vi "DecodeTriggerSettings.vi"(8 "error in (no error)":errorcluster, 9 "ParameterLabel":string, 10 "Arg":string, 11 "Highland T564 DDG in":refnum<class "Highland T564 DDG.lvclass">) -> (0 "error out":errorcluster, 3 "Highland T564 DDG out":refnum<class "Highland T564 DDG.lvclass">)   [LabVIEW 2020, in "Highland T564 DDG.lvclass"]
uses:
  Highland T564 DDG.lvclass
  C:/GEECS/Developers Version/source/Device Drivers/shared/MetaDriver_v1/MetaDriver_v1.lvclass
  shared/Typdefs/Choice81.ctl
  shared/Typdefs/Choice82.ctl
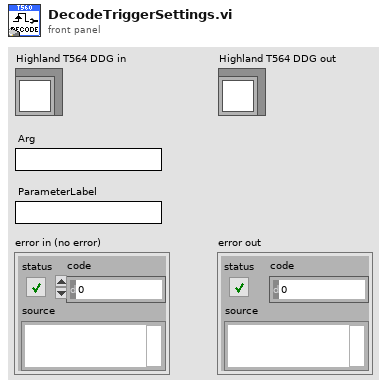
[diagram p1: front panel]
types:
  T1 = typedef "Choice81.ctl" = enum16{"10KOhm", "50Ohms"}
  T2 = typedef "Choice82.ctl" = enum16{"Rising", "Falling", "Internal 80MHz", "Internal DDS", "Remote", "Disabled"}
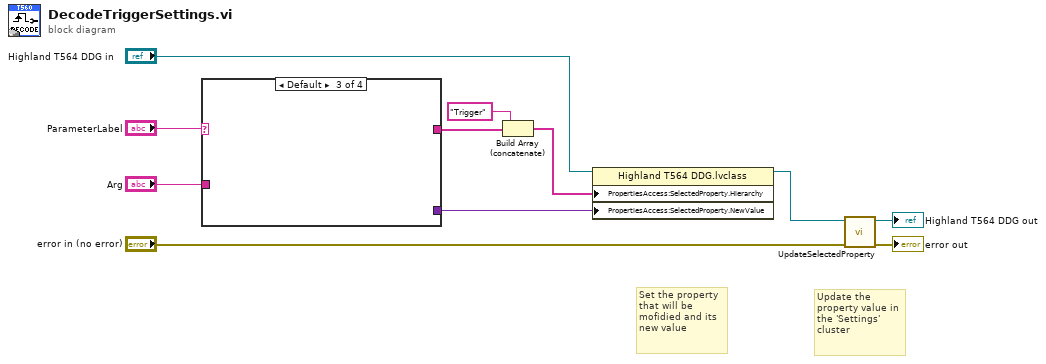
[diagram p0: block diagram]
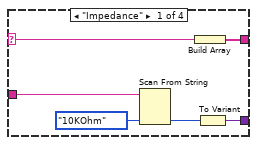
[diagram p2: hidden frame]
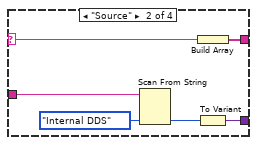
[diagram p3: hidden frame]
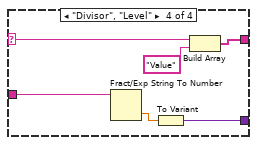
[diagram p4: hidden frame]
diagram:
  # "Update the property value in the 'Settings' cluster"
  # "Set the property that will be mofidied and its new value"
  n1 = case shown="Default" "ParameterLabel" {
    selector: "ParameterLabel" -> [w17 w23 _ w26]
    tunnel: "Arg" -> [w15 w21 _ w29]
    tunnel: [w13 w19 _ w28] -> w5
    tunnel: [w12 w18 _ w24] -> w11
    frame "Impedance" {
      n2 = Scan From String(input string=w15, default 1=Choice81."10KOhm" ("Polarity")) -> (output 1=w14:T1)  [unwired: 3 in, 3 out]
      n3 = Build Array(w17) -> (w12:string[])
      n4 = To Variant(anything=w14) -> (Variant=w13:variant)
    }
    frame "Source" {
      n5 = Scan From String(input string=w21, default 1=Choice82."Internal DDS" ("ON/OFF")) -> (output 1=w20:T2)  [unwired: 3 in, 3 out]
      n6 = Build Array(w23) -> (w18:string[])
      n7 = To Variant(anything=w20) -> (Variant=w19:variant)
    }
    frame Default {
    }
    frame "Divisor", "Level" {
      n8 = Fract/Exp String To Number(string=w29) -> (number=w27:dbl)  [unwired: 3 in, 1 out]
      n9 = To Variant(anything=w27) -> (Variant=w28:variant)
      n10 = Build Array(w26, "Value" ("element")) -> (w24:string[])
    }
  }
  n11 = Build Array (concatenate)("Trigger" ("element"), w11) -> (w6:string[])
  n12 = property class="Highland T564 DDG.lvclass"(reference="Highland T564 DDG in", "PropertiesAccess:SelectedProperty.Hierarchy"=w6, "PropertiesAccess:SelectedProperty.NewValue"=w5) -> (reference out=w2:refnum<class "Highland T564 DDG.lvclass">)  [unwired: 1 in, 1 out]
  n13 = call-dynamic "UpdateSelectedProperty.vi"("error in (no error)"="error in (no error)", "Highland T564 DDG in"=w2) -> ("error out"=→"error out":errorcluster, "Highland T564 DDG out"=→"Highland T564 DDG out":refnum<class "Highland T564 DDG.lvclass">)  [unwired: 8 in]
